vi "get header mclb.vi"(8 "error in (no error)":errorcluster, 10 "Control label":string, 11 "VI (Caller)":refnum<vi>) -> (0 "error out":errorcluster, 3 "headers":string)   [LabVIEW 2020, in "ui-testing.lvlib"]
uses:
  ui-testing.lvlib
  <vilib>/addons/Tools/Unicode/UTF8 Tools.lvlib
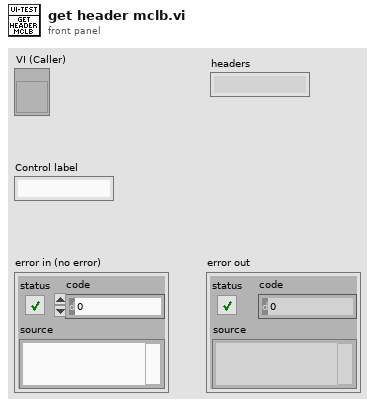
[diagram p1: front panel]
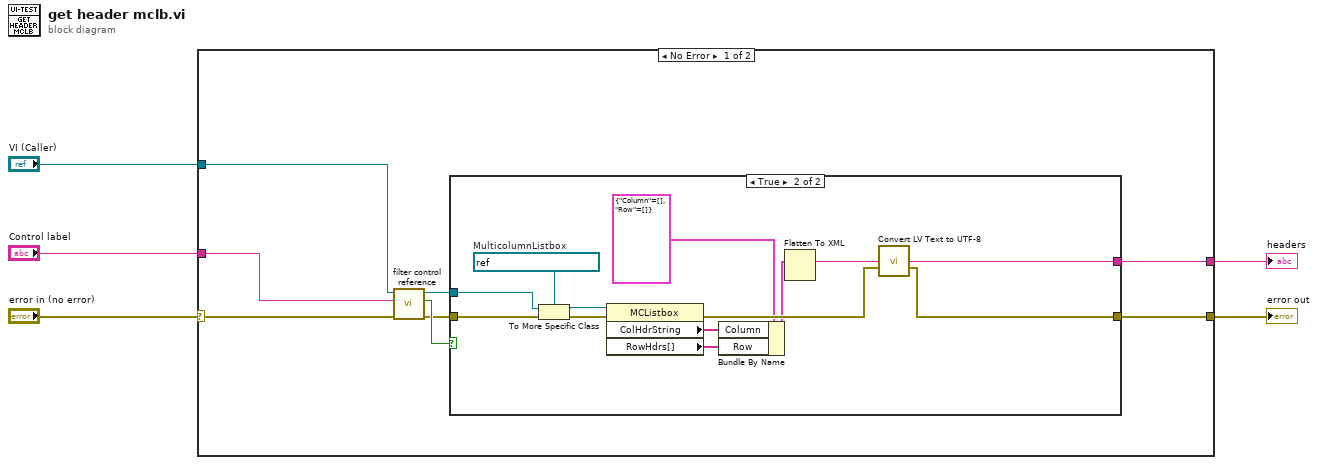
[diagram p0: block diagram]
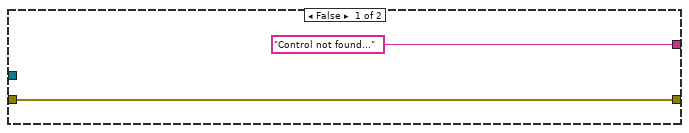
[diagram p2: hidden frame]
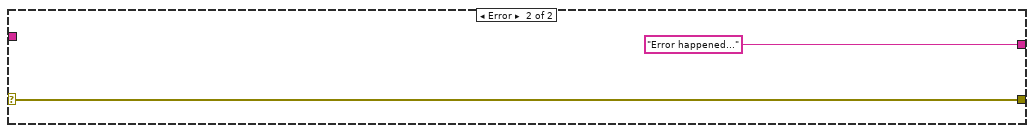
[diagram p3: hidden frame]
diagram:
  n1 = case shown="No Error" "error in (no error)" {
    selector: "error in (no error)" -> [w10 w30]
    tunnel: "Control label" -> [w9 _]
    tunnel: "VI (Caller)" -> [w8 _]
    tunnel: [w7 "Error happened..."] -> w2
    tunnel: [w6 w30] -> w1
    frame No Error {
      n2 = call "filter control reference.vi"("error in (no error)"=w10, "Control label"=w9, "VI (Caller)"=w8) -> ("error out"=w12:errorcluster, "Control found"=w13:bool, "Control ref"=w11:refnum<vi>)  [unwired: 6 in]
      n3 = case shown="True" w13 {
        tunnel: w12 -> [w15 w28]
        tunnel: w11 -> [_ w25]
        tunnel: ["Control not found..." w21] -> w7
        tunnel: [w15 w20] -> w6
        frame False {
        }
        frame True {
          w24 = refnum<vi> refnum  # MulticolumnListbox
          n4 = To More Specific Class(target class=w24, reference=w25, error in=w28) -> (specific class reference=w26:refnum<vi>, error out=w27:errorcluster)
          n5 = property class="MCListbox"(reference=w26, error in=w27) -> (error out=w22:errorcluster, "ColHdrString"=w17:string[], "RowHdrs[]"=w16:string[])  [unwired: 1 out]
          n6 = Bundle By Name(cluster=cluster{"Column":string[], "Row":string[]} {"Column"=[], "Row"=[]}, "Column"=w17, "Row"=w16) -> (w18:cluster{"Column":string[], "Row":string[]})
          n7 = Flatten To XML(6:w18) -> (2:w23:string)
          n8 = call <vilib>:"Convert LV Text to UTF-8.vi"("LV Text"=w23, "error in"=w22) -> ("UTF-8 Text"=w21:string, "error out"=w20:errorcluster)  [unwired: 12 in]
        }
      }
    }
    frame Error {
    }
  }
  "error out" <- w1
  "headers" <- w2
